vi "Quad Ctr (subVI).vi"(1 "Reset":bool, 3 "Input B":bool, 4 "Input A":bool) -> (0 "16-bit Count":u16)   [LabVIEW 2015]
doc: "This is a subVI to support a quadrature counter. It takes input from both the A Input and B Input lines of the encoder and outputs an increment or decrement of the total quadrature count. It also uses an asychronous input to reset the quadrature count.\n\nThe count is stored as an unsigned 8-bit number. It will roll over to 0 after the count of 255."
panel:
  # "This is a subVI to support a quadrature counter.  It takes input from two boolean controls and outputs an increment or decrement that represents a total quadrature count.  It also uses an asychronous input to reset the quadrature count."
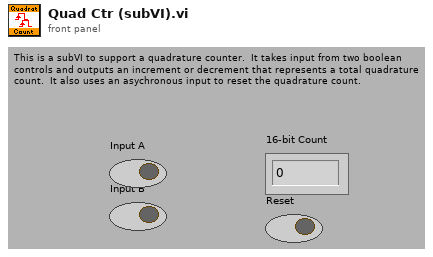
[diagram p1: front panel]
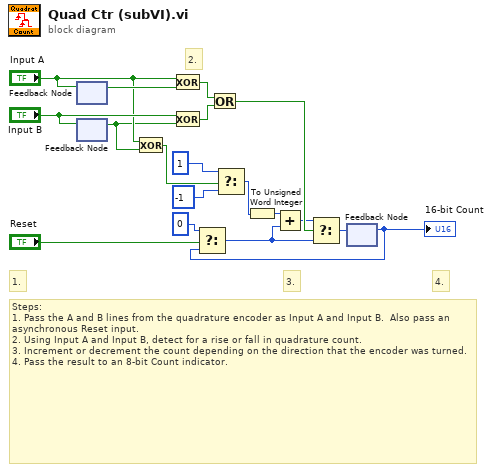
[diagram p0: block diagram]
diagram:
  # "4."
  # "3."
  # "2."
  # "1."
  # "Steps:\n1. Pass the A and B lines from the quadrature encoder as Input A and Input B.  Also pass an asynchronous Reset input.\n2. Using Input A and Input B, detect for a rise or fall in quadrature count.\n3. Increment or decrement the count depending on the direction that the encoder was turned.\n4. Pass the result to an 8-bit Count indicator."
  n1 = feedback-in #1("Input A") -> ()
  n2 = feedback #1() -> (w7:bool)  [unwired: 1 out]
  n3 = feedback-in #2("Input B") -> ()
  n4 = feedback #2() -> (w5:bool)  [unwired: 1 out]
  n5 = Exclusive Or(1:w5, 2:"Input A") -> (0:w18:bool)
  n6 = Exclusive Or(1:w7, 2:"Input A") -> (0:w16:bool)
  n7 = Exclusive Or(1:w5, 2:"Input B") -> (0:w15:bool)
  n8 = Or(x=w16, y=w15) -> (x .or. y?=w17:bool)
  n9 = Select(t=i16 1, s=w18, f=i16 -1) -> (s? t:f=w2:i16)
  n10 = To Unsigned Word Integer(number=w2) -> (unsigned 16bit integer=w3:u16)
  n11 = feedback #3() -> (w1:u16)  [unwired: 1 out]
  "16-bit Count" <- w1
  n12 = Select(t=u16 0, s="Reset", f=w1) -> (s? t:f=w11:u16)
  n13 = Add(x=w3, y=w11) -> (x+y=w9:u16)
  n14 = Select(t=w9, s=w17, f=w11) -> (s? t:f=w4:u16)
  n15 = feedback-in #3(w4) -> ()
